vi "test_output_freq_host.vi"() -> ()   [LabVIEW 2013]
uses:
  <vilib>/userdefined/High Color/nirio_resource_hc.ctl
  Config/FPGAref_config.ctl
  <vilib>/FPGAPlugInAG/PXIe-7975R/niLvFpga_Open_PXIe-7975R.vi
  <vilib>/rvi/interface/common/dynamic/niFpgaDynamicAddResources.vi
  <vilib>/rvi/interface/common/niFpgaWaitOnOcc.vi
  <vilib>/Utility/error.llb/Error Cluster From Error Code.vi
  <vilib>/rvi/errors/niLvFpgaAdjustHostInterfaceError.vi
  <vilib>/FPGAPlugInAG/Dynamic/niLvFpga_Close_Dynamic.vi
  <vilib>/rvi/interface/nirviOpenFPGA/nirviOpenFPGA.xnode
  FPGA Bitfiles/mixer_FPGATarget2_testoutputfreqfp_S+JHlaCnIjM.lvbitx
  FPGA/test_output_freq_fpga.vi
  <vilib>/rvi/interface/nirviReadWriteControl/nirviReadWriteControl.xnode
  <vilib>/rvi/interface/nirviCloseFPGA/nirviCloseFPGA.xnode
  NiFpgaLv.dll
  <vilib>/rvi/interface/Simulation/niFpgaSimulationCallBeginRW.vi
panel:
  in  "stop":bool
  in  "samples per period":fxp<+,32,32>=50000000.0
  out "error out":errorcluster
  in  "resource name":T1="RIO0"
  out "Clocking Option Configured?":bool
  out "Configured?":bool
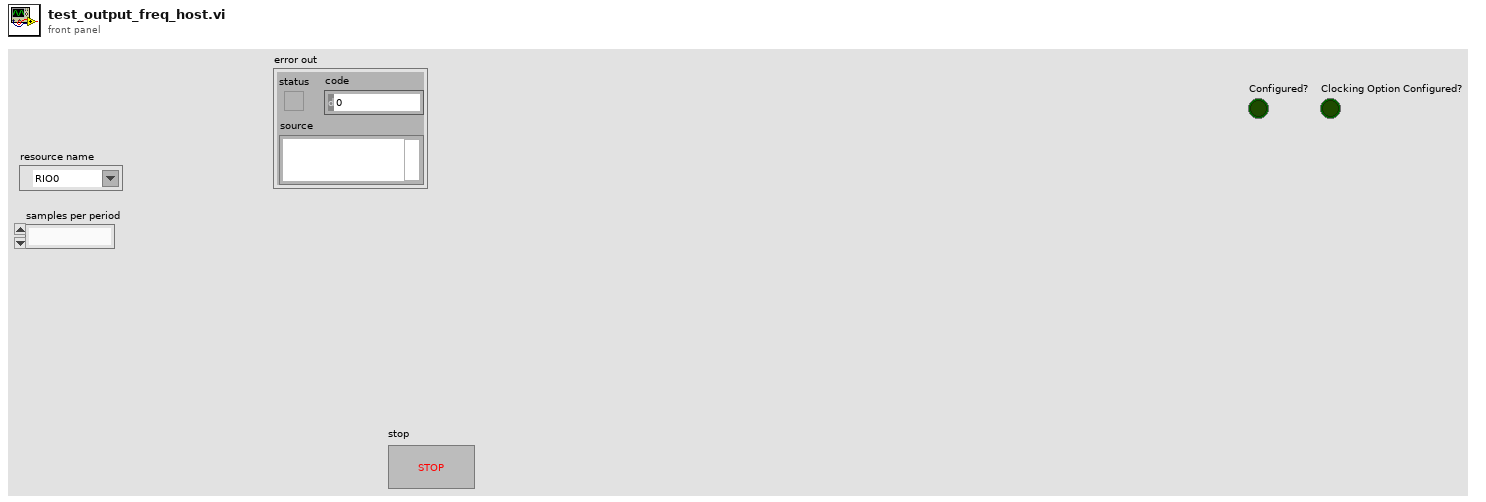
[diagram p1: front panel]
types:
  T1 = typedef "nirio_resource_hc.ctl" = tag
  T2 = typedef "FPGAref_config.ctl" = refnum<k20>
  T3 = enum8{"Internal Clock PLL Off", "Internal Clock PLL On (REF IN)", "External Clock (CLK_IN)", "Internal Clock PLL On (IoModSyncClk)"}
  T4 = typedef "FPGAref_5782.ctl" = refnum<k20>
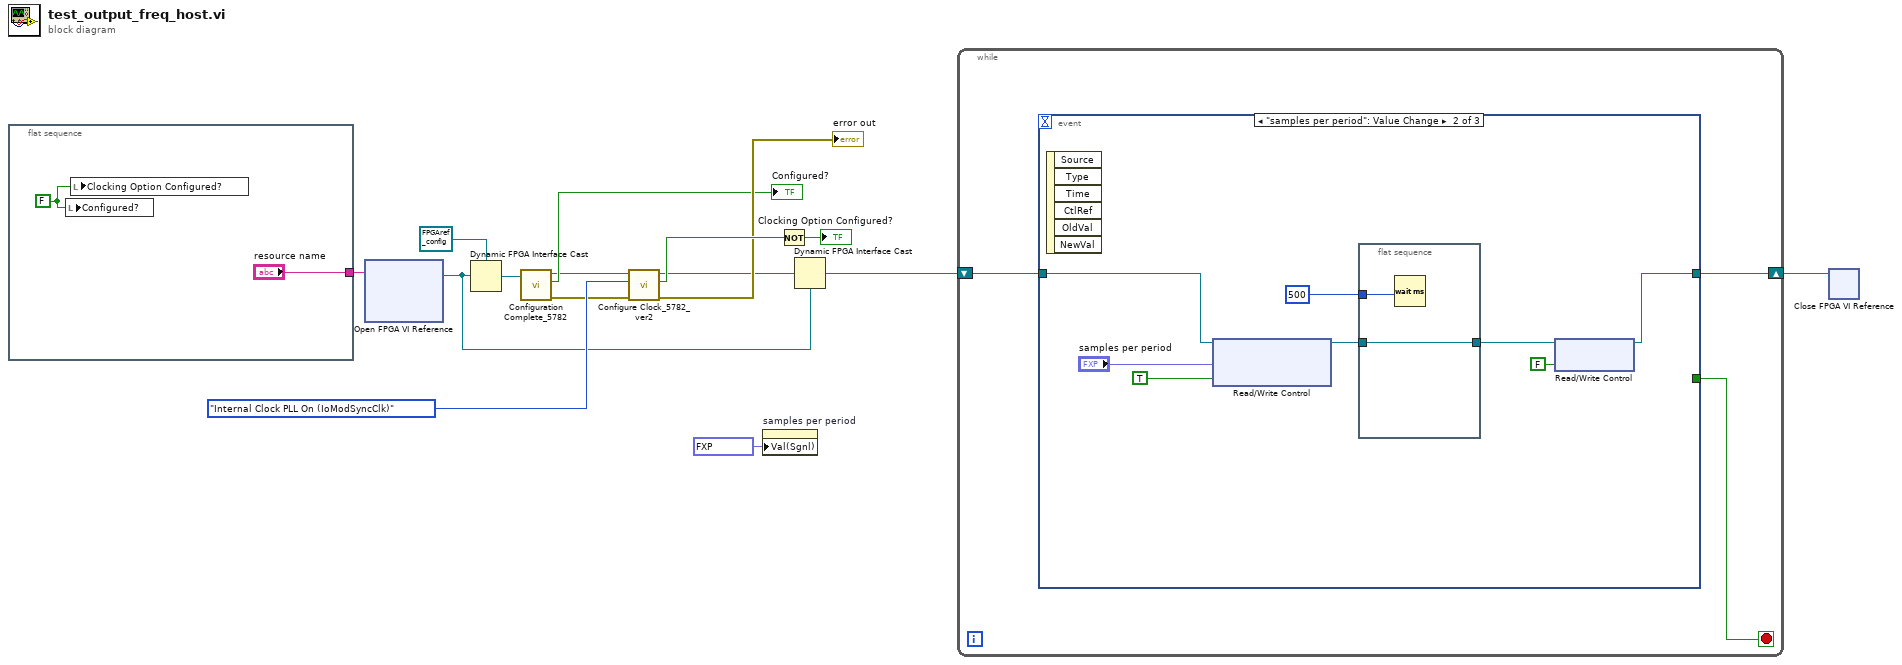
[diagram p0: block diagram]
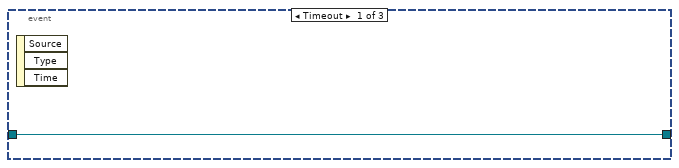
[diagram p2: hidden frame]
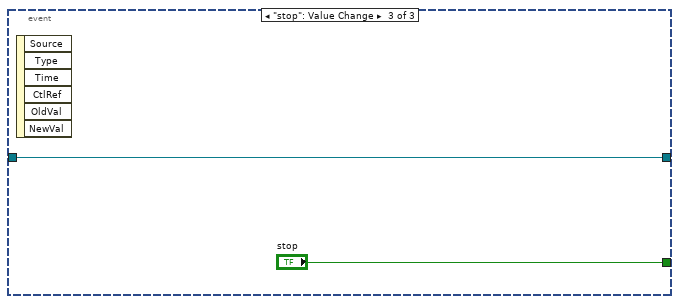
[diagram p3: hidden frame]
diagram:
  n1 = flat-sequence {
    tunnel: ["resource name"] -> w14
    frame #0 {
      w16 = FALSE ("Trigger Acquisition")
      n2 = local write "Configured?"(w16) -> ()
      n3 = local write "Clocking Option Configured?"(w16) -> ()
    }
  }
  n4 = xnode "Open FPGA VI Reference"("resource name"=w14) -> ("FPGA VI Reference Out"=w5:refnum<k20>)  [unwired: 1 in, 1 out]
  n5 = Dynamic FPGA Interface Cast(Session In=T2 refnum ("FPGA VI Reference in"), Type=w5) -> (Session Out=w6:T2)
  n6 = call "Configuration Complete_5782.vi"("FPGA VI Reference in"=w6) -> ("error out"=w9:errorcluster, "Configured?"=→"Configured?":bool, "FPGA VI Reference Out"=w8:T4)  [unwired: 8 in]
  n7 = call "Configure Clock_5782_ver2.vi"("error in"=w9, "Clock Source"=T3."Internal Clock PLL On (IoModSyncClk)", "FPGA VI Reference"=w8) -> ("error out"=→"error out":errorcluster, "Configuration Error"=w12:bool, "FPGA VI Reference Out"=w4:T4)  [unwired: 6 in]
  n8 = property on="samples per period" class="DigNum (strict)"("Val(Sgnl)"=fxp<+,32,32> 500000000.0 ("Value (Signaling)")) -> ()  [unwired: 2 in, 2 out]
  n9 = Not(x=w12) -> (.not. x?=→"Clocking Option Configured?":bool)
  n10 = Dynamic FPGA Interface Cast(Session In=w5, Type=w4) -> (Session Out=w3:refnum<k20>)
  n11 = while {
    shift-right: [w18] -> w1
    shift-left: w3 -> [w20]
    stop <- w19 stop-if-true
    n12 = event shown="[1] \"samples per period\": Value Change" {
      selector: _ -> [_ _ _]
      dyn-events: _ -> [_ _ _]
      timeout: _ -> [_ _ _]
      tunnel: w20 -> [w21 w23 w32]
      tunnel: [_ _ "stop"] -> w19
      tunnel: [w21 w22 w32] -> w18
      event Timeout {
        n13 = event-data() -> ()  [unwired: 1 in, 3 out]
      }
      event "samples per period": Value Change {
        n14 = event-data() -> ()  [unwired: 1 in, 6 out]
        n15 = xnode "Read/Write Control"("FPGA VI Reference In"=w23, "samples per period"="samples per period", "set samples"=TRUE) -> ("FPGA VI Reference Out"=w27:refnum<k20>)  [unwired: 1 in, 1 out]
        n16 = flat-sequence {
          tunnel: w27 -> [w30]
          tunnel: u32 500 ("milliseconds to wait") -> [w31]
          tunnel: [w30] -> w25
          frame #0 {
            n17 = Wait (ms)(milliseconds to wait=w31) -> ()  [unwired: 1 out]
          }
        }
        n18 = xnode "Read/Write Control"("FPGA VI Reference In"=w25, "set samples"=FALSE) -> ("FPGA VI Reference Out"=w22:refnum<k20>)  [unwired: 1 in, 1 out]
      }
      event "stop": Value Change {
        n19 = event-data() -> ()  [unwired: 1 in, 6 out]
      }
    }
  }
  n20 = xnode "Close FPGA VI Reference"("FPGA VI Reference In"=w1) -> ()  [unwired: 1 in, 1 out]
